vi "Legacy Detector.vi"(7 "Unit ID (A)":string="A", 8 "error in":errorcluster, 11 "VISA Session In":refnum<visa-resource-name>="Alicat") -> (0 "error out":errorcluster, 2 "Legacy Status":u8(ring) items=["Rev. 21 Board", "Rev. 22 Board", "Rev. 23 Board"], 3 "VISA Session Out":refnum<visa-resource-name>)   [LabVIEW 2024]
doc: "Returns the revision of the circuit board that the Alicat contains. This is used to determine whether certain features and functiona are available using other Alicat sub-VI's."
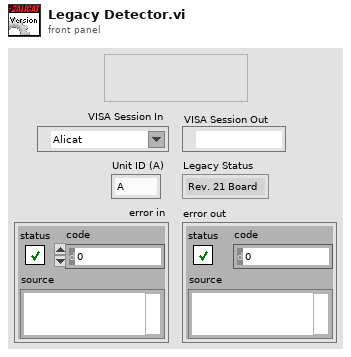
[diagram p1: front panel]
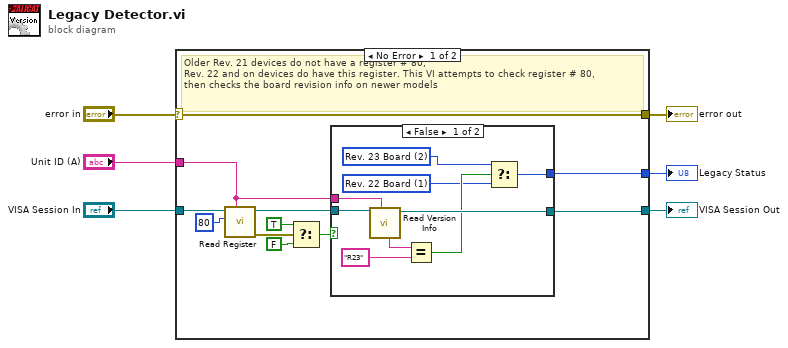
[diagram p0: block diagram]
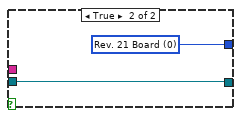
[diagram p2: hidden frame]
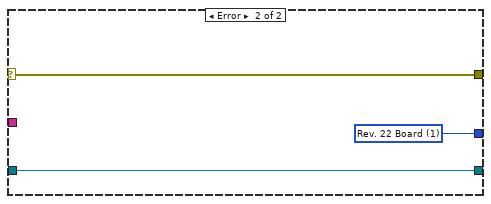
[diagram p3: hidden frame]
diagram:
  n1 = case shown="No Error" "error in" {
    selector: "error in" -> [w12 w30]
    tunnel: [w12 w30] -> w5
    tunnel: "VISA Session In" -> [w11 w31]
    tunnel: "Unit ID (A)" -> [w7 _]
    tunnel: [w9 w31] -> w2
    tunnel: [w8 w29] -> w1
    frame No Error {
      # "Older Rev. 21 devices do not have a register # 80,\nRev. 22 and on devices do have this register. This VI attempts to check register # 80,\nthen checks the board revision info on newer models"
      n2 = call "Read Register.vi"("Unit ID (A)"=w7, "Register address"=u16 80, "VISA Session In"=w11) -> ("error out"=w16:errorcluster, "VISA Session Out"=w10:refnum<visa-resource-name>)  [unwired: 6 in, 1 out]
      n3 = Select(t=TRUE, s=w16, f=FALSE) -> (s? t:f=w13:bool)
      n4 = case shown="False" w13 {
        tunnel: [w19 w28] -> w8
        tunnel: w10 -> [w26 w27]
        tunnel: [w23 w27] -> w9
        tunnel: w7 -> [w18 _]
        frame False {
          w20 = u8 1 items=["Rev. 21 Board", "Rev. 22 Board", "Rev. 23 Board"] ("Legacy Status")
          w21 = u8 2 items=["Rev. 21 Board", "Rev. 22 Board", "Rev. 23 Board"] ("Legacy Status")
          n5 = call "Read Version Info.vi"("Unit ID (A)"=w18, "VISA Session In"=w26) -> ("VISA Session Out"=w23:refnum<visa-resource-name>, "Board Rev"=w25:string)  [unwired: 5 in, 3 out]
          n6 = Equal?(x=w25, y="R23" ("x")) -> (x = y?=w22:bool)
          n7 = Select(t=w21, s=w22, f=w20) -> (s? t:f=w19:u8)
        }
        frame True {
          w28 = u8 0 items=["Rev. 21 Board", "Rev. 22 Board", "Rev. 23 Board"] ("Legacy Status")
        }
      }
    }
    frame Error {
      w29 = u8 1 items=["Rev. 21 Board", "Rev. 22 Board", "Rev. 23 Board"] ("Legacy Status")
    }
  }
  "error out" <- w5
  "VISA Session Out" <- w2
  "Legacy Status" <- w1
